vi "Add HTTP Route.vi"(8 "error in (no error)":errorcluster, 10 "Nav Route":refnum<class "Nav Route.lvclass">, 11 "VolatusAPI in":refnum<class "VolatusAPI.lvclass">) -> (0 "error out":errorcluster, 3 "VolatusAPI out":refnum<class "VolatusAPI.lvclass">)   [LabVIEW 2020, in "Volatus.lvlib" / "VolatusAPI.lvclass"]
uses:
  VolatusAPI.lvclass
  Nav Route/Nav Route.lvclass
  VolatusAPI.lvclass/VolatusAPI.ctl
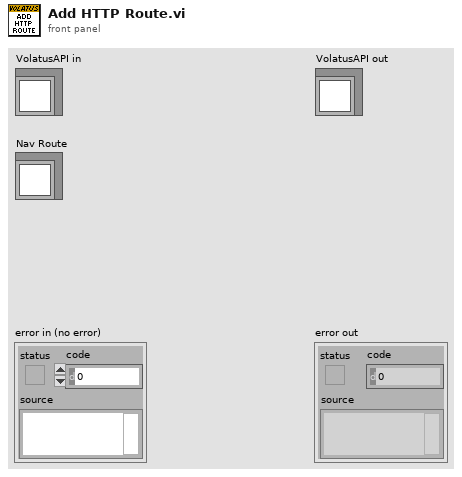
[diagram p1: front panel]
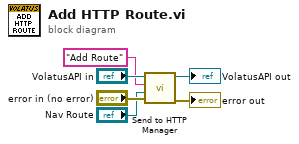
[diagram p0: block diagram]
diagram:
  n1 = call "Send to HTTP Manager.vi"("error in (no error)"="error in (no error)", "Data"="Nav Route", "ID"="Add Route", "VolatusAPI in"="VolatusAPI in") -> ("error out"=→"error out":errorcluster, "VolatusAPI out"=→"VolatusAPI out":refnum<class "VolatusAPI.lvclass">)  [unwired: 6 in]
